vi "Config.vi"(0 "User Trigger":bool, 1 "error in":errorcluster) -> (2 "Config":u32[](array[numeric]), 3 "All Config Data":string[][](array[string]), 4 "error out":errorcluster)   [LabVIEW 2018]
uses:
  <vilib>/Utility/file.llb/Write Delimited Spreadsheet (string).vi
  <vilib>/Utility/file.llb/Read Delimited Spreadsheet (string).vi
panel:
  in  "Update":bool
  in  "Anchor Fore":bool
  in  "Mast Fore":bool
  in  "Manuvering Light":bool
  in  "Stern":bool
  in  "Mast Aft":bool
  in  "Anchor Aft":bool
  in  "Side Light  Port":bool
  in  "Side Light STBD":bool
  in  "Condition Name":string
  in  "Clear All":bool
  in  "Remove":bool
  in  "Add":bool
  in  "Special Condition":i32(listbox)
  in  "Lamp Selection":enum16{"1", "2"}(ring)
  in  "Power Supply":enum16{"2", "1"}(ring)
  in  "Save Button":bool
  in  "Lamp Selection Mode":enum16{"Manual", "Auto"}(ring)
  in  "Power Supply Mode":enum16{"Manual", "Auto"}(ring)
  # "CONFIGURE NLCS"
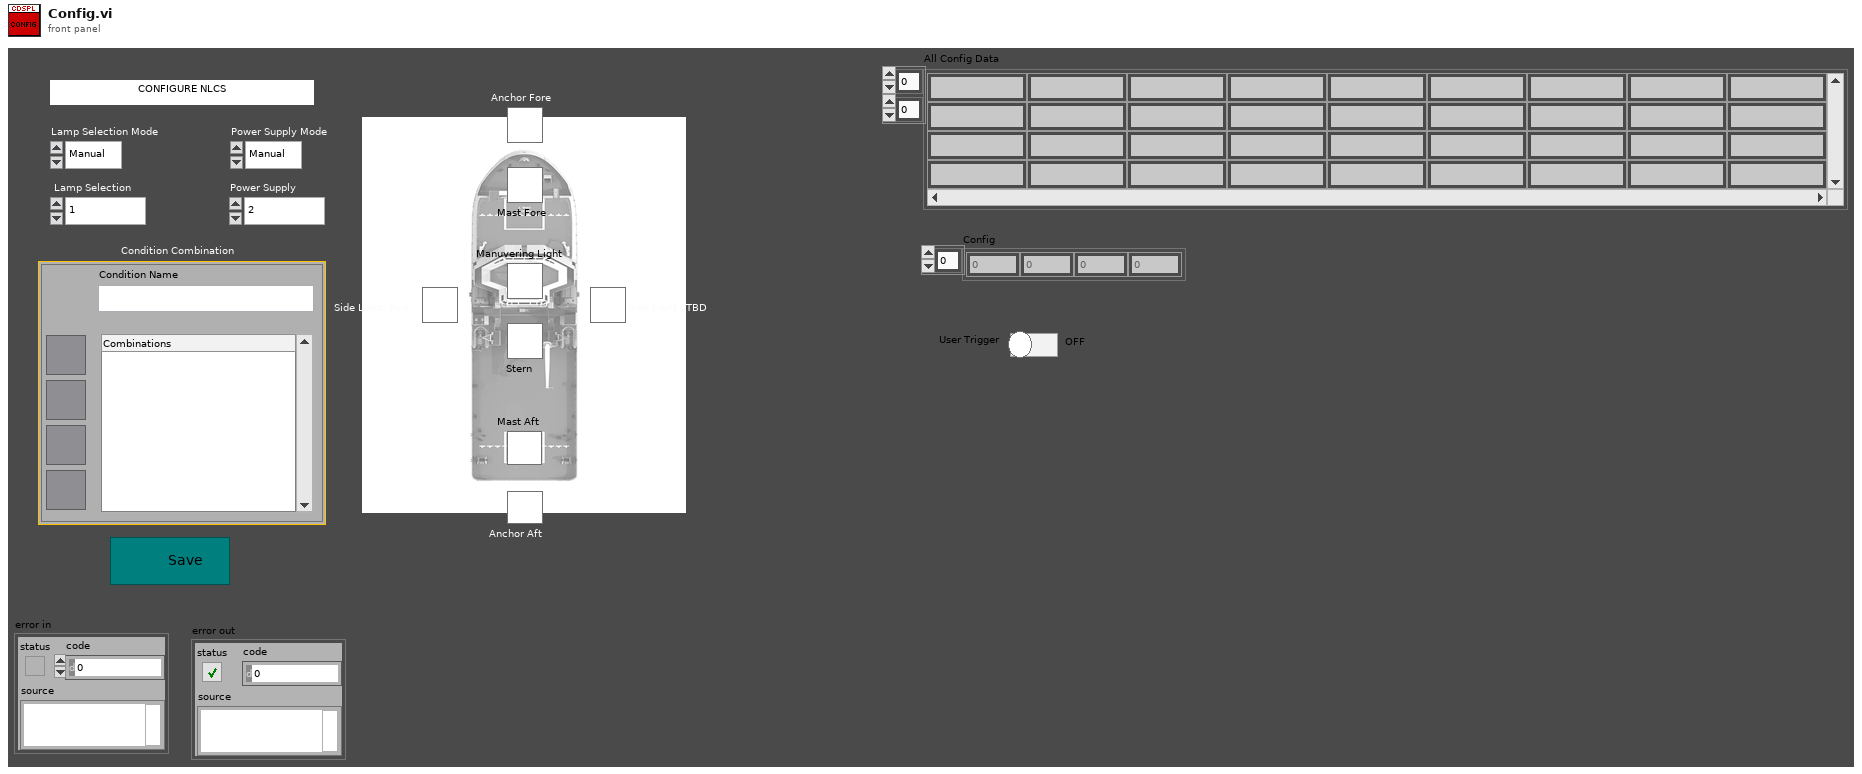
[diagram p1: front panel]
types:
  T1 = enum8{"Enabled", "Disabled", "Disabled and Grayed Out"}
  T2 = enum32{"Invalid", "Standard", "Closed", "Hidden", "Minimized", "Maximized"}
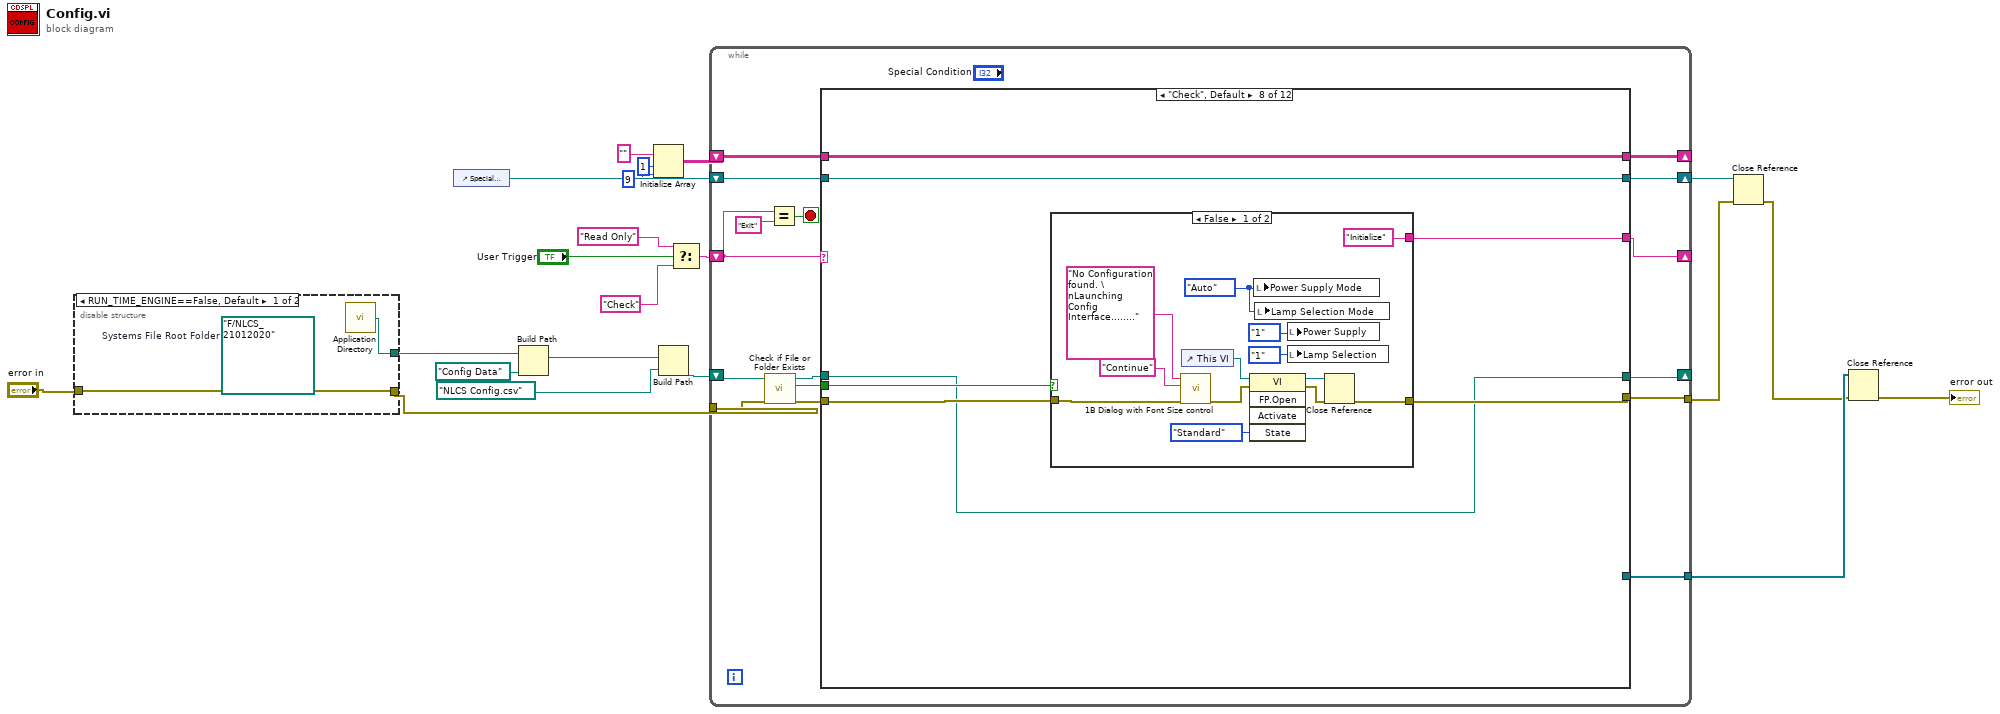
[diagram p0: block diagram]
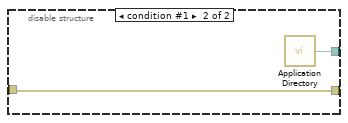
[diagram p2: hidden frame]
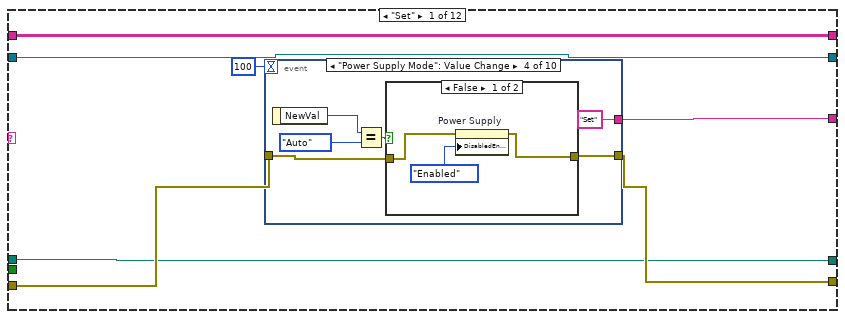
[diagram p3: hidden frame]
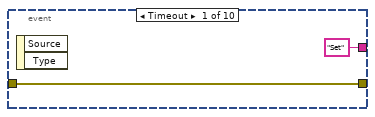
[diagram p4: hidden frame]
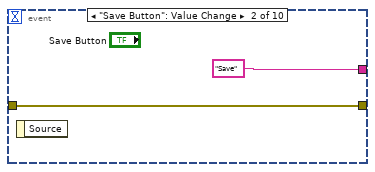
[diagram p5: hidden frame]
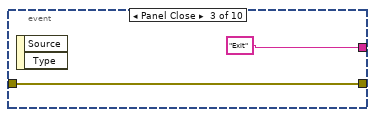
[diagram p6: hidden frame]
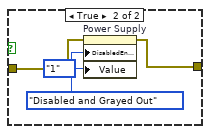
[diagram p7: hidden frame]
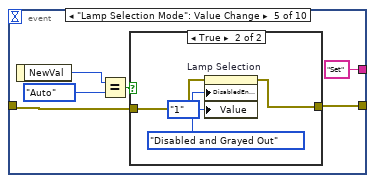
[diagram p8: hidden frame]
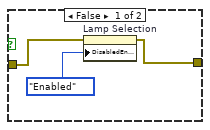
[diagram p9: hidden frame]
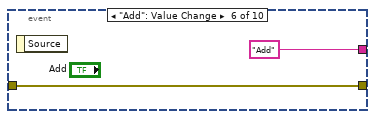
[diagram p10: hidden frame]
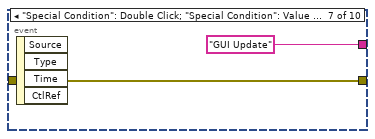
[diagram p11: hidden frame]
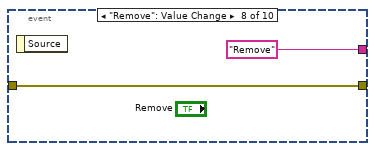
[diagram p12: hidden frame]
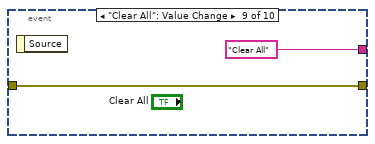
[diagram p13: hidden frame]
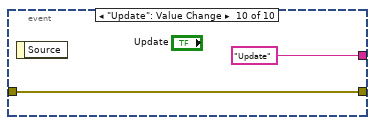
[diagram p14: hidden frame]
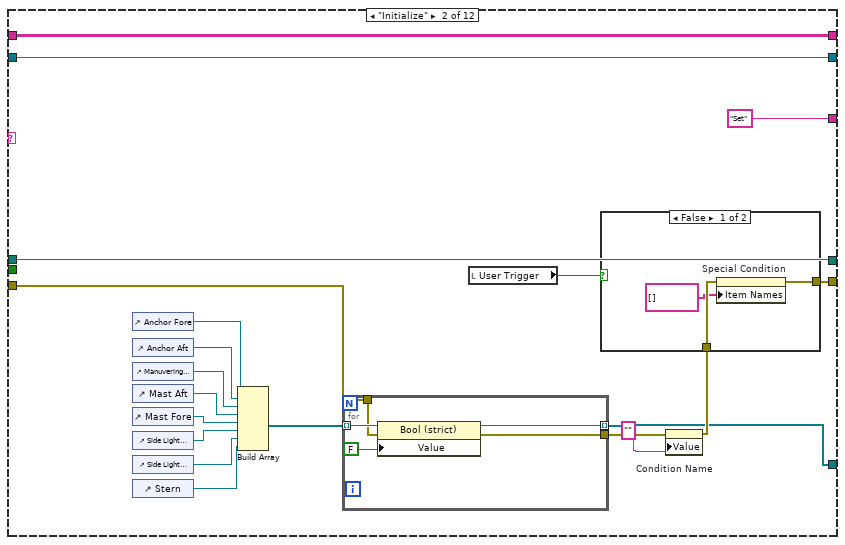
[diagram p15: hidden frame]
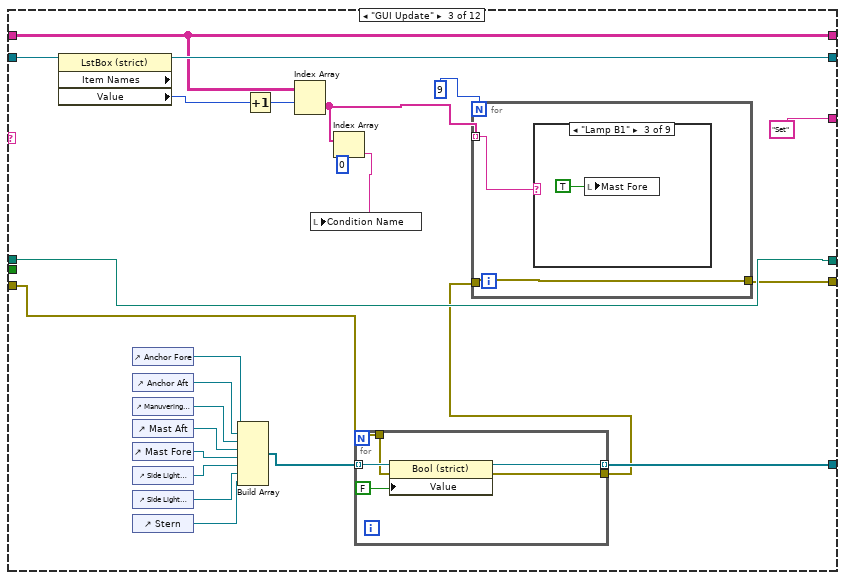
[diagram p17: hidden frame]
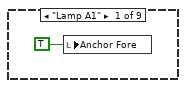
[diagram p18: hidden frame]
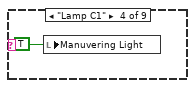
[diagram p20: hidden frame]
diagram:
  n1 = disable-structure shown="RUN_TIME_ENGINE==False, Default" {
    disable-tunnel: [w22 w25] -> w11
    disable-tunnel: [w23 w24] -> w17
    disable-tunnel: "error in" -> [w23 w24]
    frame condition #0 (active) {
      (unwired) path "F:/NLCS_21012020"  # Systems File Root Folder
      n2 = call <vilib>:"Application Directory.vi"() -> ("Application Directory"=w22:path)
    }
    frame condition #1 {
      n3 = call <vilib>:"Application Directory.vi"() -> ("Application Directory"=w25:path)
    }
  }
  n4 = control-ref of="Special Condition"() -> (w10:refnum<vi>)
  n5 = Build Path(base path=w11, name or relative path=path "Config Data" ("default name")) -> (appended path=w20:path)
  n6 = Initialize Array("", 1 ("dimension size"), 9 ("dimension size")) -> (w6:string[][])
  n7 = Build Path(base path=w20, name or relative path=path "NLCS Config.csv" ("default name")) -> (appended path=w19:path)
  n8 = Select(t="Read Only" ("y"), s="User Trigger", f="Check" ("y")) -> (s? t:f=w12:string)
  n9 = while {
    shift-right: [w31] -> _
    shift-left: w12 -> [w33]
    tunnel: w17 -> [w37]
    shift-right: [w40] -> _
    shift-left: w19 -> [w39]
    tunnel: [w41] -> w8
    shift-right: [w29] -> _
    shift-left: w6 -> [w30]
    shift-right: [w27] -> w9
    shift-left: w10 -> [w28]
    tunnel: [w26] -> w4
    stop <- w32 stop-if-true
    n10 = call <vilib>:"Check if File or Folder Exists.vi"("error in (no error)"=w37, "path"=w39) -> ("error out"=w35:errorcluster, "file or folder exists?"=w36:bool, "dup path"=w38:path)  [unwired: 7 in]
    n11 = Equal?(x=w33, y="Exit") -> (x = y?=w32:bool)
    n12 = case shown="\"Check\", Default" w33 {
      tunnel: [w45 "Set" ("y") "Set" ("y") "Set" ("y") "Set" ("y") "Set" ("y") "Set" ("y") w304 "Read" "Exit" "Initialize" "Exit"] -> w31
      tunnel: w38 -> [w46 w100 w141 w179 w239 w276 w287 w301 w346 w377 w400 w430]
      tunnel: w35 -> [w48 w101 w130 _ _ w277 w286 w303 w341 w384 w410 w428]
      tunnel: [w47 w93 w127 w180 w240 w277 w286 w302 w347 w383 w404 w427] -> w41
      tunnel: [w46 w100 w141 w179 w239 w276 w287 w301 w344 w376 w399 w430] -> w40
      tunnel: w36 -> [_ _ _ _ _ _ _ w305 w342 _ _ _]
      tunnel: w30 -> [w44 w98 w126 w164 w222 w272 w294 w300 w333 w380 _ w426]
      tunnel: [w44 w98 w126 w181 w241 w279 w295 w300 w332 w380 w390 w426] -> w29
      tunnel: w28 -> [w43 w99 w143 w182 w242 w281 w298 w299 w334 w379 w401 w425]
      tunnel: [w43 w99 w142 w178 w238 w280 w288 w299 w334 w379 w401 w425] -> w27
      tunnel: [_ w92 w129 _ _ _ _ _ _ _ _ _] -> w26
      frame "Set" {
        n13 = event shown="[3] \"Power Supply Mode\": Value Change" {
          selector: _ -> [_ _ _ _ _ _ _ _ _ _]
          dyn-events: _ -> [_ _ _ _ _ _ _ _ _ _]
          timeout: 100 -> [_ _ _ _ _ _ _ _ _ _]
          tunnel: ["Set" "Save" "Exit" "Set" "Set" "Add" "GUI Update" "Remove" "Clear All" "Update"] -> w45
          tunnel: w48 -> [w50 w51 w53 w57 w70 w81 w83 w86 w87 w89]
          tunnel: [w50 w51 w53 w56 w69 w81 w83 w86 w87 w89] -> w47
          event Timeout {
            n14 = event-data() -> ()  [unwired: 1 in, 2 out]
          }
          event "Save Button": Value Change {
            n15 = event-data() -> ()  [unwired: 1 in, 1 out]
          }
          event Panel Close {
            n16 = event-data() -> ()  [unwired: 1 in, 2 out]
          }
          event "Power Supply Mode": Value Change {
            n17 = event-data() -> ("NewVal"=w60:enum16{"Manual", "Auto"})  [unwired: 1 in]
            n18 = Equal?(x=w60, y=enum16{"Manual", "Auto"}."Auto" ("Lamp Selection Mode")) -> (x = y?=w58:bool)
            n19 = case shown="False" w58 {
              tunnel: w57 -> [w62 w67]
              tunnel: [w61 w66] -> w56
              frame False {
                n20 = property on="Power Supply" class="Enum (strict)"(error in=w62, "DisabledEnum"=T1."Enabled" ("Disabled")) -> (error out=w61:errorcluster)  [unwired: 1 in, 1 out]
              }
              frame True {
                n21 = property on="Power Supply" class="Enum (strict)"(error in=w67, "DisabledEnum"=T1."Disabled and Grayed Out" ("Disabled"), "Value"=enum16{"2", "1"}."1" ("Power Supply")) -> (error out=w66:errorcluster)  [unwired: 1 in, 1 out]
              }
            }
          }
          event "Lamp Selection Mode": Value Change {
            n22 = event-data() -> ("NewVal"=w73:enum16{"Manual", "Auto"})  [unwired: 1 in]
            n23 = Equal?(x=w73, y=enum16{"Manual", "Auto"}."Auto" ("Lamp Selection Mode")) -> (x = y?=w71:bool)
            n24 = case shown="True" w71 {
              tunnel: w70 -> [w75 w80]
              tunnel: [w74 w79] -> w69
              frame False {
                n25 = property on="Lamp Selection" class="Enum (strict)"(error in=w75, "DisabledEnum"=T1."Enabled" ("Disabled")) -> (error out=w74:errorcluster)  [unwired: 1 in, 1 out]
              }
              frame True {
                n26 = property on="Lamp Selection" class="Enum (strict)"(error in=w80, "DisabledEnum"=T1."Disabled and Grayed Out" ("Disabled"), "Value"=enum16{"1", "2"}."1" ("Lamp Selection")) -> (error out=w79:errorcluster)  [unwired: 1 in, 1 out]
              }
            }
          }
          event "Add": Value Change {
            n27 = event-data() -> ()  [unwired: 1 in, 1 out]
          }
          event "Special Condition": Double Click; "Special Condition": Value Change {
            n28 = event-data() -> ()  [unwired: 1 in, 4 out]
          }
          event "Remove": Value Change {
            n29 = event-data() -> ()  [unwired: 1 in, 1 out]
          }
          event "Clear All": Value Change {
            n30 = event-data() -> ()  [unwired: 1 in, 1 out]
          }
          event "Update": Value Change {
            n31 = event-data() -> ()  [unwired: 1 in, 1 out]
          }
        }
      }
      frame "Initialize" {
        n32 = control-ref of="Anchor Fore"() -> (w110:refnum<vi>)
        n33 = control-ref of="Anchor Aft"() -> (w109:refnum<vi>)
        n34 = control-ref of="Manuvering Light"() -> (w108:refnum<vi>)
        n35 = control-ref of="Mast Aft"() -> (w107:refnum<vi>)
        n36 = control-ref of="Mast Fore"() -> (w106:refnum<vi>)
        n37 = control-ref of="Side Light  Port"() -> (w105:refnum<vi>)
        n38 = control-ref of="Side Light STBD"() -> (w104:refnum<vi>)
        n39 = control-ref of="Stern"() -> (w103:refnum<vi>)
        n40 = Build Array(w110, w109, w108, w107, w106, w105, w104, w103) -> (w102:refnum<vi>[])
        n41 = for {
          tunnel: w102 -> [w119] mode=indexing
          tunnel: w101 -> [w117]
          tunnel: [w116] -> w97
          tunnel: [w115] -> w92 mode=indexing
          n42 = property class="Bool (strict)"(reference=w119, error in=w117, "Value"=FALSE) -> (reference out=w115:refnum<vi>, error out=w116:errorcluster)
        }
        n43 = local read "User Trigger"() -> (w91:bool)
        n44 = property on="Condition Name" class="Str"(error in=w97, "Value"="" ("Condition Name")) -> (error out=w94:errorcluster)  [unwired: 1 in, 1 out]
        n45 = case shown="False" w91 {
          tunnel: w94 -> [w113 w114]
          tunnel: [w112 w114] -> w93
          frame False {
            n46 = property on="Special Condition" class="LstBox (strict)"(error in=w113, "Item Names"=string[] []) -> (error out=w112:errorcluster)  [unwired: 1 in, 1 out]
          }
          frame True {
          }
        }
      }
      frame "GUI Update" {
        n47 = property on="Property Node" class="LstBox (strict)" props=["Item Names", "Value"](reference=w143) -> (reference out=w142:refnum<vi>, "Value"=w124:i32)  [unwired: 1 in, 2 out]
        n48 = control-ref of="Anchor Fore"() -> (w139:refnum<vi>)
        n49 = control-ref of="Anchor Aft"() -> (w138:refnum<vi>)
        n50 = control-ref of="Manuvering Light"() -> (w137:refnum<vi>)
        n51 = control-ref of="Mast Aft"() -> (w136:refnum<vi>)
        n52 = control-ref of="Mast Fore"() -> (w135:refnum<vi>)
        n53 = control-ref of="Side Light  Port"() -> (w134:refnum<vi>)
        n54 = control-ref of="Side Light STBD"() -> (w133:refnum<vi>)
        n55 = control-ref of="Stern"() -> (w132:refnum<vi>)
        n56 = Build Array(w139, w138, w137, w136, w135, w134, w133, w132) -> (w131:refnum<vi>[])
        n57 = Increment(x=w124) -> (x+1=w123:i32)
        n58 = Index Array(array=w126, index (row)=w123) -> (element=w122:string[])  [unwired: 1 in]
        n59 = Index Array(array=w122, index=0) -> (element=w120:string)
        n60 = local write "Condition Name"(w120) -> ()
        n61 = for {
          tunnel: w131 -> [w148] mode=indexing
          tunnel: w130 -> [w146]
          tunnel: [w145] -> w128
          tunnel: [w144] -> w129 mode=indexing
          n62 = property class="Bool (strict)"(reference=w148, error in=w146, "Value"=FALSE) -> (reference out=w144:refnum<vi>, error out=w145:errorcluster)
        }
        n63 = for {
          N: 9 -> [_]
          tunnel: w122 -> [w150] mode=indexing
          tunnel: w128 -> [w149]
          tunnel: [w149] -> w127
          n64 = case shown="\"Lamp B1\"" w150 {
            frame "Lamp A1" {
              n65 = local write "Anchor Fore"(TRUE ("Anchor Fore")) -> ()
            }
            frame Default {
            }
            frame "Lamp B1" {
              n66 = local write "Mast Fore"(TRUE ("Mast Fore")) -> ()
            }
            frame "Lamp C1" {
              n67 = local write "Manuvering Light"(TRUE ("Manuvering Light")) -> ()
            }
            frame "Lamp D1" {
              n68 = local write "Stern"(TRUE ("Stern")) -> ()
            }
            frame "Lamp E1" {
              n69 = local write "Mast Aft"(TRUE ("Mast Aft")) -> ()
            }
            frame "Lamp F1" {
              n70 = local write "Anchor Aft"(TRUE ("Anchor Aft")) -> ()
            }
            frame "Lamp G1" {
              n71 = local write "Side Light  Port"(TRUE ("Side Light  Port")) -> ()
            }
            frame "Lamp H1" {
              n72 = local write "Side Light STBD"(TRUE ("Side Light STBD")) -> ()
            }
          }
        }
      }
      frame "Add" {
        n73 = while {
          tunnel: ["Lamp A1"] -> w170 if="Anchor Fore"
          tunnel: ["Lamp B1"] -> w171 if="Mast Fore"
          tunnel: ["Lamp C1"] -> w172 if="Manuvering Light"
          tunnel: ["Lamp D1"] -> w173 if="Stern"
          tunnel: ["Lamp E1"] -> w174 if="Mast Aft"
          tunnel: ["Lamp F1"] -> w175 if="Anchor Aft"
          tunnel: ["Lamp G1"] -> w176 if="Side Light  Port"
          tunnel: ["Lamp H1"] -> w177 if="Side Light STBD"
          stop <- TRUE stop-if-true
        }
        n74 = property on="Property Node" class="LstBox (strict)"(reference=w182) -> (reference out=w183:refnum<vi>, error out=w184:errorcluster, "Item Names"=w163:string[], "Value"=w161:i32)  [unwired: 1 in]
        n75 = Increment(x=w161) -> (x+1=w162:i32)
        n76 = Array Size(array=w163) -> (size(s)=w186:i32)
        n77 = case shown="0, Default" w186 {
          tunnel: [w213 w216] -> w185
          tunnel: w163 -> [w214 w218]
          tunnel: "Condition Name" -> [w212 w217]
          tunnel: w162 -> [w211 w215]
          tunnel: [w211 w215] -> w159
          frame 0, Default {
            n78 = Build Array (concatenate)(w214, w212) -> (w213:string[])
          }
          frame 1.. {
            n79 = Insert Into Array(array=w218, index=w215, new element=w217) -> (w216:string[])
          }
        }
        n80 = Build Array(w170, w171, w172, w173, w174, w175, w176, w177) -> (w166:string[])
        n81 = property on="Property Node" class="LstBox (strict)"(reference=w183, error in=w184, "Item Names"=w185, "Value"=w162) -> (reference out=w178:refnum<vi>, error out=w180:errorcluster)
        n82 = for {
          N: 8 -> [_]
          shift-right: [w193] -> w165
          shift-left: w166 -> [w189]
          stop <- w190 stop-if-true
          n83 = Search 1D Array(1D array=w189, element="") -> (index of element=w191:i32)  [unwired: 1 in]
          n84 = Less Than 0?(x=w191) -> (x < 0?=w190:bool)
          n85 = Delete From Array(array=w189, length=1 ("index"), index=w191) -> (array with subset deleted=w193:string[])  [unwired: 1 out]
        }
        n86 = Build Array (concatenate)("Condition Name", w165) -> (w168:string[])
        n87 = Increment(x=w159) -> (x+1=w160:i32)
        n88 = Insert Into Array(array=w164, index (row)=w160, new element=w168) -> (w181:string[][])  [unwired: 1 in]
      }
      frame "Update" {
        n89 = local read "Condition Name"() -> (w224:string)
        n90 = while {
          tunnel: ["Lamp A1"] -> w230 if=w260
          tunnel: ["Lamp B1"] -> w231 if=w253
          tunnel: ["Lamp C1"] -> w232 if=w254
          tunnel: ["Lamp D1"] -> w233 if=w255
          tunnel: ["Lamp E1"] -> w234 if=w256
          tunnel: ["Lamp F1"] -> w235 if=w257
          tunnel: ["Lamp G1"] -> w236 if=w258
          tunnel: ["Lamp H1"] -> w237 if=w259
          stop <- TRUE stop-if-true
          n91 = local read "Manuvering Light"() -> (w254:bool)
          n92 = local read "Side Light STBD"() -> (w259:bool)
          n93 = local read "Side Light  Port"() -> (w258:bool)
          n94 = local read "Anchor Fore"() -> (w260:bool)
          n95 = local read "Anchor Aft"() -> (w257:bool)
          n96 = local read "Mast Fore"() -> (w253:bool)
          n97 = local read "Mast Aft"() -> (w256:bool)
          n98 = local read "Stern"() -> (w255:bool)
        }
        n99 = property on="Property Node" class="LstBox (strict)"(reference=w242) -> (reference out=w243:refnum<vi>, error out=w244:errorcluster, "Item Names"=w225:string[], "Value"=w223:i32)  [unwired: 1 in]
        n100 = Replace Array Subset(array=w225, new element=w224, index=w223) -> (w245:string[])
        n101 = Build Array(w230, w231, w232, w233, w234, w235, w236, w237) -> (w227:string[])
        n102 = property on="Property Node" class="LstBox (strict)"(reference=w243, error in=w244, "Item Names"=w245) -> (reference out=w238:refnum<vi>, error out=w240:errorcluster)
        n103 = for {
          N: 8 -> [_]
          shift-right: [w252] -> w226
          shift-left: w227 -> [w248]
          stop <- w249 stop-if-true
          n104 = Search 1D Array(1D array=w248, element="") -> (index of element=w250:i32)  [unwired: 1 in]
          n105 = Less Than 0?(x=w250) -> (x < 0?=w249:bool)
          n106 = Delete From Array(array=w248, length=1 ("index"), index=w250) -> (array with subset deleted=w252:string[])  [unwired: 1 out]
        }
        n107 = Build Array (concatenate)(w224, w226) -> (w229:string[])
        n108 = Increment(x=w223) -> (x+1=w221:i32)
        n109 = Delete From Array(array=w222, length=1, index (row)=w221) -> (array with subset deleted=w219:string[][])  [unwired: 1 in, 1 out]
        n110 = Insert Into Array(array=w219, index (row)=w221, new element=w229) -> (w241:string[][])  [unwired: 1 in]
      }
      frame "Remove" {
        n111 = property on="Property Node" class="LstBox (strict)"(reference=w281) -> (reference out=w285:refnum<vi>, error out=w284:errorcluster, "Item Names"=w274:string[], "Value"=w271:i32)  [unwired: 1 in]
        n112 = Delete From Array(array=w274, length=1, index=w271) -> (array with subset deleted=w282:string[])  [unwired: 1 out]
        n113 = Decrement(x=w271) -> (x-1=w275:i32)
        n114 = property on="Property Node" class="LstBox (strict)"(reference=w285, error in=w284, "Item Names"=w282, "Value"=w275) -> (reference out=w280:refnum<vi>)  [unwired: 1 out]
        n115 = Increment(x=w271) -> (x+1=w270:i32)
        n116 = Delete From Array(array=w272, length=1, index (row)=w270) -> (array with subset deleted=w279:string[][])  [unwired: 1 in, 1 out]
      }
      frame "Clear All" {
        n117 = property on="Property Node" class="LstBox (strict)"(reference=w298, "Item Names"=string[] [] ("ItemNames")) -> (reference out=w288:refnum<vi>)  [unwired: 1 in, 1 out]
        n118 = Array Size(array=w294) -> (size(s)=w293:i32[])
        n119 = Index Array(array=w293, index=0) -> (element=w291:i32)
        n120 = Decrement(x=w291) -> (x-1=w290:i32)
        n121 = Delete From Array(array=w294, length=w290, index (row)=0) -> (array with subset deleted=w295:string[][])  [unwired: 1 in, 1 out]
      }
      frame "Check", Default {
        n122 = case shown="False" w305 {
          tunnel: ["Initialize" ("y") "Read" ("y")] -> w304
          tunnel: w303 -> [w317 w320]
          tunnel: [w310 w319] -> w302
          frame False {
            w308 = enum16{"Manual", "Auto"}."Auto" ("Power Supply Mode")
            n123 = call "1B Dialog with Font Size control.vi"("error in (no error)"=w317, "T Button Name (\"OK\")"="Continue" ("button name (\"OK\")"), "message"="No Configuration found. \nLaunching Config Interface........") -> ("error out"=w311:errorcluster)  [unwired: 7 in, 1 out]
            n124 = control-ref of="This VI"() -> (w309:refnum<vi>)
            n125 = invoke class="VI" method="FP.Open"(reference=w309, error in=w311, "State"=T2."Standard") -> (reference out=w314:refnum<vi>, error out=w313:errorcluster)  [unwired: 2 in, 3 out]
            n126 = local write "Power Supply Mode"(w308) -> ()
            n127 = local write "Lamp Selection Mode"(w308) -> ()
            n128 = local write "Power Supply"(enum16{"2", "1"}."1" ("Power Supply")) -> ()
            n129 = local write "Lamp Selection"(enum16{"1", "2"}."1" ("Lamp Selection")) -> ()
            n130 = Close Reference(reference=w314, error in (no error)=w313) -> (error out=w310:errorcluster)
          }
          frame True {
            n131 = disable-structure shown="Enabled" {
              disable-tunnel: w320 -> [w323 w330]
              disable-tunnel: [w322 w330] -> w319
              frame Enabled {
                n132 = Current VI's Path() -> (path=w325:path)
                n133 = Open VI Reference(vi path=w325, error in (no error)=w323) -> (vi reference=w326:refnum<vi>, error out=w327:errorcluster)  [unwired: 4 in]
                n134 = invoke class="VI" method="FP.Open"(reference=w326, error in=w327, "State"=T2."Hidden") -> (reference out=w329:refnum<vi>, error out=w328:errorcluster)  [unwired: 2 in, 3 out]
                n135 = Close Reference(reference=w329, error in (no error)=w328) -> (error out=w322:errorcluster)
              }
              frame Disabled {
              }
            }
          }
        }
      }
      frame "Save" {
        n136 = case shown="False" w342 {
          tunnel: w346 -> [w354 w367]
          tunnel: [w353 w366] -> w345
          tunnel: [w352 w367] -> w344
          tunnel: w341 -> [w351 w366]
          frame False {
            n137 = disable-structure shown="Enabled" {
              disable-tunnel: w354 -> [w358 w362]
              disable-tunnel: [w357 w364] -> w353
              disable-tunnel: [w356 w362] -> w352
              disable-tunnel: w351 -> [w355 w365]
              frame Disabled {
                n138 = call "File Dialog"("start path"=w358, "prompt"="Save Config", "default name"="NLCS Config" ("prompt"), "error in"=w355, "pattern (all files)"="*.csv") -> ("selected path"=w356:path, "error out"=w357:errorcluster)  [unwired: 7 in, 2 out]
              }
              frame Enabled {
                n139 = Strip Path(path=w362) -> (stripped path=w363:path)  [unwired: 1 out]
                n140 = Create Folder(path (use dialog)=w363, error in=w365) -> (error out=w364:errorcluster)  [unwired: 1 in, 2 out]
              }
            }
          }
          frame True {
          }
        }
        n141 = Build Array("Power Supply Mode", "Power Supply", "Lamp Selection Mode", "Lamp Selection") -> (w336:u16[])
        n142 = for {
          tunnel: w336 -> [w350] mode=indexing
          tunnel: [w349] -> w335 mode=indexing
          n143 = Format Into String(w350) -> (resulting string=w349:string)  [unwired: 3 in, 1 out]
        }
        n144 = Replace Array Subset(array=w333, new element=w335, index (row)=0 ("index")) -> (w332:string[][])  [unwired: 1 in]
        n145 = call-poly <vilib>:"Write Delimited Spreadsheet.vi"("file path (dialog if empty)"=w344, "2D data"=w332, "error in (no error)"=w345, "transpose? (no:F)"=FALSE) -> ("error out"=w347:errorcluster)  [unwired: 10 in, 1 out]
      }
      frame "Read" {
        w369 = u32 1 ("x")
        n146 = call-poly <vilib>:"Read Delimited Spreadsheet.vi"("file path (dialog if empty)"=w377, "error in (no error)"=w384) -> ("new file path (Not A Path if cancelled)"=w376:path, "all rows"=w378:string[][], "error out"=w383:errorcluster)  [unwired: 8 in, 3 out]
        "All Config Data" <- w378
        n147 = Index Array(array=w378, index (row)=0) -> (element=w381:string[])  [unwired: 1 in]
        n148 = Octal String To Number(4:w381) -> (0:w375:u32[])  [unwired: 2 in, 1 out]
        "Config" <- w375
        n149 = Index Array(array=w375, index #1=0 ("index"), index #2=2 ("index")) -> (element #1=w372:u32, element #2=w371:u32)
        n150 = Equal?(x=w372, y=w369) -> (x = y?=w368:bool)
        n151 = Equal?(x=w369, y=w371) -> (x = y?=w370:bool)
        n152 = case shown="False" w368 {
          frame False {
          }
          frame True {
            n153 = property on="Power Supply" class="Enum (strict)"("DisabledEnum"=T1."Disabled and Grayed Out" ("Disabled"), "Value"=enum16{"2", "1"}."2" ("Power Supply")) -> ()  [unwired: 2 in, 2 out]
          }
        }
        n154 = case shown="False" w370 {
          frame False {
          }
          frame True {
            n155 = property on="Lamp Selection" class="Enum (strict)"("DisabledEnum"=T1."Disabled and Grayed Out" ("Disabled"), "Value"=enum16{"1", "2"}."1" ("Lamp Selection")) -> ()  [unwired: 2 in, 2 out]
          }
        }
      }
      frame "Read Only" {
        n156 = call-poly <vilib>:"Read Delimited Spreadsheet.vi"("file path (dialog if empty)"=w400, "error in (no error)"=w410) -> ("new file path (Not A Path if cancelled)"=w399:path, "all rows"=w390:string[][], "error out"=w395:errorcluster)  [unwired: 8 in, 3 out]
        n157 = Index Array(array=w390, index (col)=0 ("disabled index (col)")) -> (element=w396:string[])  [unwired: 1 in]
        n158 = Delete From Array(array=w396, length=1, index=0) -> (array with subset deleted=w393:string[])  [unwired: 1 out]
        n159 = control-ref of="Lamp Selection"() -> (w405:refnum<vi>)
        n160 = control-ref of="Power Supply Mode"() -> (w406:refnum<vi>)
        n161 = control-ref of="Power Supply"() -> (w402:refnum<vi>)
        n162 = control-ref of="Lamp Selection Mode"() -> (w403:refnum<vi>)
        n163 = property on="Special Condition" class="LstBox (strict)"(error in=w395, "Item Names"=w393) -> (error out=w394:errorcluster)  [unwired: 1 in, 1 out]
        n164 = Index Array(array=w390, index (row)=0) -> (element=w408:string[])  [unwired: 1 in]
        n165 = disable-structure shown="Enabled" {
          disable-tunnel: w394 -> [w414 w420]
          disable-tunnel: [w413 w420] -> w404
          frame Enabled {
            n166 = Current VI's Path() -> (path=w419:path)
            n167 = Open VI Reference(vi path=w419, error in (no error)=w414) -> (vi reference=w418:refnum<vi>, error out=w417:errorcluster)  [unwired: 4 in]
            n168 = invoke class="VI" method="FP.Open"(reference=w418, error in=w417, "State"=T2."Standard") -> (reference out=w415:refnum<vi>, error out=w416:errorcluster)  [unwired: 2 in, 3 out]
            n169 = Close Reference(reference=w415, error in (no error)=w416) -> (error out=w413:errorcluster)
          }
          frame Disabled {
          }
        }
        n170 = Build Array(w406, w402, w403, w405) -> (w407:refnum<vi>[])
        n171 = for {
          N: 4 -> [_]
          tunnel: w408 -> [w421] mode=indexing
          tunnel: w407 -> [w423] mode=indexing
          n172 = Octal String To Number(4:w421) -> (0:w422:u32)  [unwired: 2 in, 1 out]
          n173 = property class="Enum"(reference=w423, "Value"=w422) -> (reference out=w424:refnum<vi>)  [unwired: 1 in, 1 out]
          n174 = Close Reference(reference=w424) -> ()  [unwired: 1 in, 1 out]
        }
      }
      frame "Exit" {
        n175 = disable-structure shown="Enabled" {
          disable-tunnel: w428 -> [w434 w452]
          disable-tunnel: [w432 w452] -> w427
          frame Enabled {
            n176 = Current VI's Path() -> (path=w443:path)
            n177 = flat-sequence {
              tunnel: w434 -> [w450]
              tunnel: [errorcluster {"status"=FALSE, "code"=0, "source"=""} ("error out")] -> w435
              tunnel: [w450] -> w433
              frame #0 {
              }
            }
            n178 = Open VI Reference(vi path=w443, error in (no error)=w435) -> (vi reference=w439:refnum<vi>, error out=w437:errorcluster)  [unwired: 4 in]
            n179 = property class="VI"(reference=w439, error in=w437) -> (reference out=w438:refnum<vi>, error out=w436:errorcluster, "FP.State"=w440:T2)
            n180 = case shown="\"Standard\", \"Hidden\"..\"Maximized\"" w440 {
              tunnel: w438 -> [w445 w449]
              tunnel: w436 -> [w444 w448]
              tunnel: [w444 w447] -> w442
              tunnel: [w445 w446] -> w441
              frame "Invalid", "Closed", Default {
              }
              frame "Standard", "Hidden".."Maximized" {
                n181 = invoke class="VI" method="FP.Close"(reference=w449, error in=w448) -> (reference out=w446:refnum<vi>, error out=w447:errorcluster)  [unwired: 1 in, 1 out]
              }
            }
            n182 = Close Reference(reference=w441, error in (no error)=w442) -> (error out=w431:errorcluster)
            n183 = Merge Errors(w431, w433) -> (w432:errorcluster)
          }
          frame Disabled {
          }
        }
      }
    }
  }
  n184 = Close Reference(reference=w9, error in (no error)=w8) -> (error out=w3:errorcluster)
  n185 = Close Reference(reference=w4, error in (no error)=w3) -> (error out=→"error out":errorcluster)
